vi "tm_trans.vi"(10 "Long":dbl, 11 "Lat":dbl) -> (2 "Numeric":dbl, 3 "out_pt":dbl)   [LabVIEW 2020]
uses:
  <vilib>/imath/engines/lvmath2/RunTimeEngine/Managers/WorkSpace/UID Generator.vi
  <vilib>/imath/engines/lvmath2/RunTimeEngine/RunTimeType/NIMS_RunTimeType_From StrictType (excl LVString).vi
  <instcachedir>/0/NIMS_RunTimeType_From StrictType (excl LVString)_283B1B2000484AAA8744D21CE97EA49F.lvgen/NIMS_RunTimeType_From StrictType (excl LVString)_283B1B2000484AAA8744D21CE97EA49F_000.vi
  <vilib>/imath/engines/lvmath2/RunTimeEngine/LocalVariableDefStatement/MC_LocalVariableDefStatement_Display.vi
  <vilib>/imath/engines/lvmath2/RunTimeEngine/Managers/SymbolTable/Clear UID.vi
  <vilib>/imath/engines/lvmath2/RunTimeEngine/NodeEndStatement/NIMS_NodeEndStatement_Output.vi
  <instcachedir>/0/NIMS_NodeEndStatement_Output_53EC0D466D134D7ABD903AC30B43404B.lvgen/NIMS_NodeEndStatement_Output_53EC0D466D134D7ABD903AC30B43404B_001.vi
  <vilib>/imath/engines/lvmath2/RunTimeEngine/ErrorHandling/NIMS_Finalize Error.vi
  <vilib>/imath/engines/lvmath2/RunTimeEngine/Managers/SymbolTable/NIMS_WorkSpace.lvlib
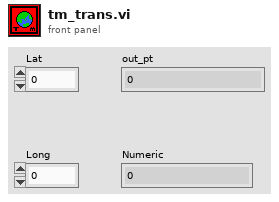
[diagram p1: front panel]
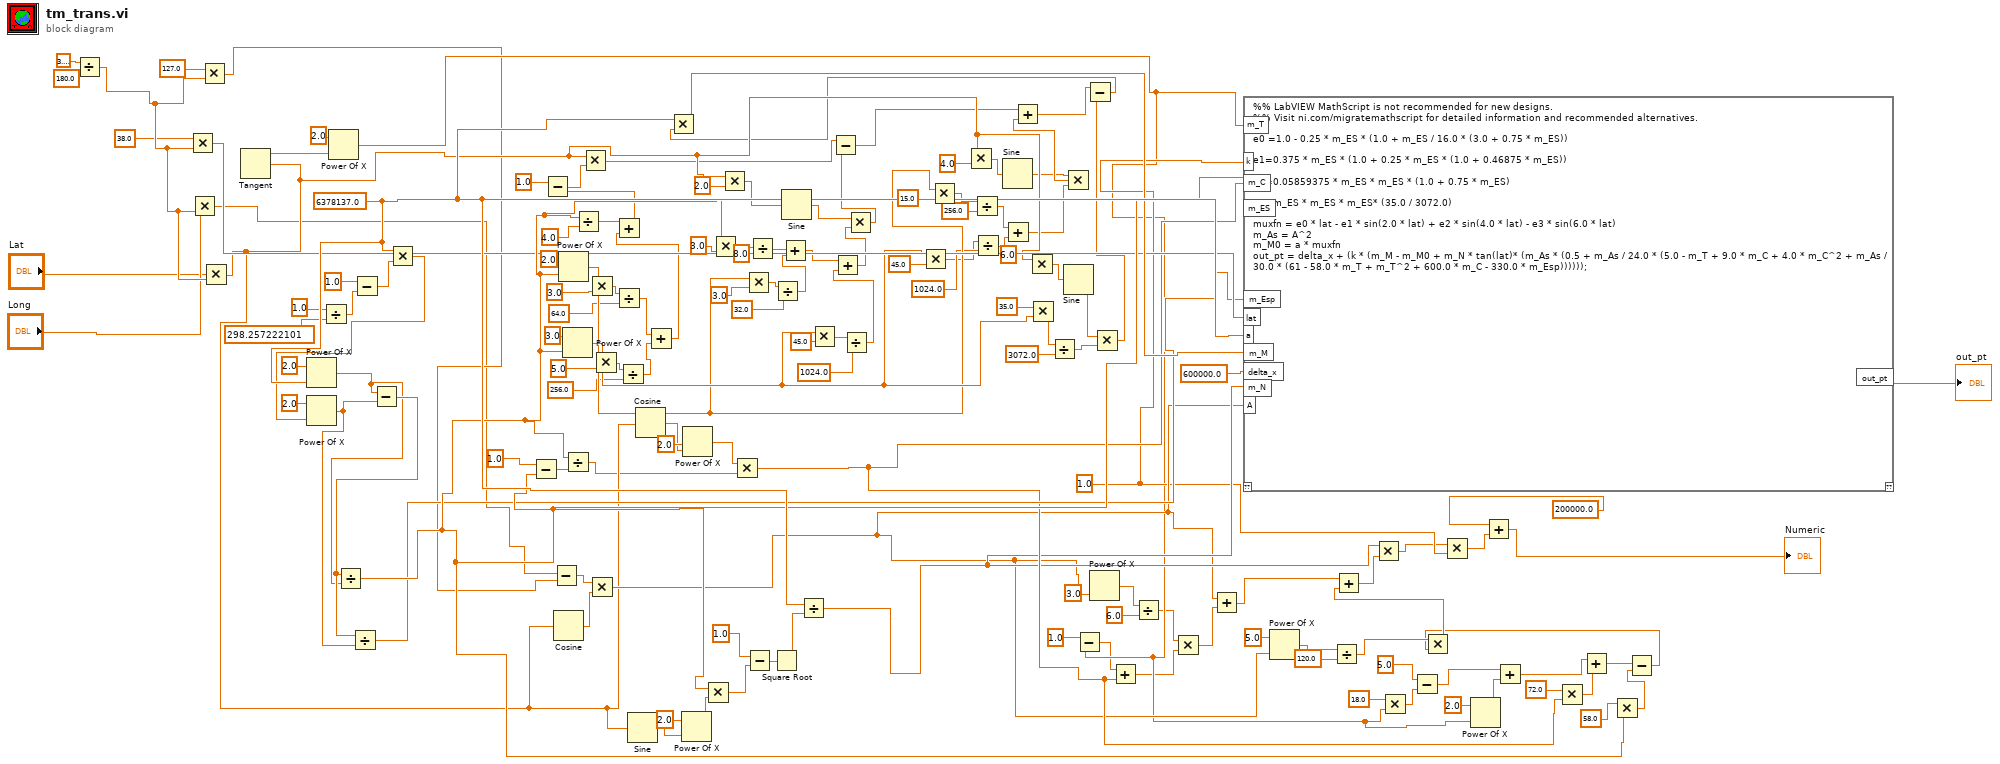
[diagram p0: block diagram]
diagram:
  w133 = 1.0 ("k")
  w143 = 6378137.0
  n1 = Divide(x=3.141592653589793, y=180.0) -> (x/y=w127:dbl)
  n2 = Multiply(x=38.0 ("Latitude0"), y=w127) -> (x*y=w140:dbl)
  n3 = Multiply(x="Long", y=w127) -> (x*y=w129:dbl)
  n4 = Multiply(x=127.0 ("Longtitude0"), y=w127) -> (x*y=w130:dbl)
  n5 = Multiply(x="Lat", y=w127) -> (x*y=w131:dbl)
  n6 = Tangent(1:w131) -> (0:w11:dbl)
  n7 = Power Of X(1:w143, 2:2.0 ("y")) -> (0:w88:dbl)
  n8 = Divide(x=1.0, y=298.257222101) -> (x/y=w6:dbl)
  n9 = Power Of X(1:w11, 2:2.0 ("x")) -> (0:w132:dbl)
  n10 = Subtract(x=1.0, y=w6) -> (x-y=w9:dbl)
  n11 = Multiply(x=w143, y=w9) -> (x*y=w128:dbl)
  n12 = Power Of X(1:w128, 2:2.0 ("y")) -> (0:w90:dbl)
  n13 = Subtract(x=w88, y=w90) -> (x-y=w89:dbl)
  n14 = Divide(x=w89, y=w88) -> (x/y=w141:dbl)
  n15 = Divide(x=w89, y=w90) -> (x/y=w139:dbl)
  n16 = Subtract(x=1.0, y=w141) -> (x-y=w74:dbl)
  n17 = Subtract(x=w129, y=w130) -> (x-y=w80:dbl)
  n18 = Cosine(x=w131) -> (cos(x)=w79:dbl)
  n19 = Power Of X(1:w141, 2:2.0 ("y")) -> (0:w91:dbl)
  n20 = Power Of X(1:w141, 2:3.0 ("y")) -> (0:w92:dbl)
  n21 = Divide(x=w141, y=w74) -> (x/y=w78:dbl)
  n22 = Divide(x=w141, y=4.0) -> (x/y=w26:dbl)
  n23 = Multiply(x=w91, y=3.0) -> (x*y=w17:dbl)
  n24 = Multiply(x=w80, y=w79) -> (x*y=w134:dbl)
  n25 = Multiply(x=w92, y=5.0) -> (x*y=w21:dbl)
  n26 = Divide(x=w17, y=64.0) -> (x/y=w24:dbl)
  n27 = Divide(x=w21, y=256.0) -> (x/y=w23:dbl)
  n28 = Sine(x=w131) -> (sin(x)=w83:dbl)
  n29 = Cosine(x=w131) -> (cos(x)=w75:dbl)
  n30 = Add(x=w24, y=w23) -> (x+y=w25:dbl)
  n31 = Add(x=w26, y=w25) -> (x+y=w27:dbl)
  n32 = Subtract(x=1.0, y=w27) -> (x-y=w29:dbl)
  n33 = Multiply(x=w131, y=w29) -> (x*y=w47:dbl)
  n34 = Power Of X(1:w83, 2:2.0 ("y")) -> (0:w85:dbl)
  n35 = Power Of X(1:w75, 2:2.0 ("y")) -> (0:w77:dbl)
  n36 = Multiply(x=w141, y=w85) -> (x*y=w86:dbl)
  n37 = Multiply(x=w141, y=3.0) -> (x*y=w31:dbl)
  n38 = Multiply(x=w131, y=2.0) -> (x*y=w44:dbl)
  n39 = Multiply(x=w77, y=w78) -> (x*y=w136:dbl)
  n40 = Multiply(x=w91, y=3.0) -> (x*y=w34:dbl)
  n41 = Subtract(x=1.0, y=w86) -> (x-y=w81:dbl)
  n42 = Divide(x=w31, y=8.0) -> (x/y=w37:dbl)
  n43 = Square Root(x=w81) -> (sqrt(x)=w87:dbl)
  n44 = Divide(x=w34, y=32.0) -> (x/y=w36:dbl)
  n45 = Add(x=w37, y=w36) -> (x+y=w42:dbl)
  n46 = Sine(x=w44) -> (sin(x)=w46:dbl)
  n47 = Divide(x=w143, y=w87) -> (x/y=w135:dbl)
  n48 = Multiply(x=w92, y=45.0) -> (x*y=w40:dbl)
  n49 = Divide(x=w40, y=1024.0) -> (x/y=w41:dbl)
  n50 = Add(x=w42, y=w41) -> (x+y=w45:dbl)
  n51 = Multiply(x=w46, y=w45) -> (x*y=w48:dbl)
  n52 = Subtract(x=w47, y=w48) -> (x-y=w61:dbl)
  n53 = Multiply(x=w92, y=45.0) -> (x*y=w53:dbl)
  n54 = Multiply(x=w91, y=15.0) -> (x*y=w50:dbl)
  n55 = Multiply(x=w131, y=4.0) -> (x*y=w58:dbl)
  n56 = Divide(x=w50, y=256.0) -> (x/y=w55:dbl)
  n57 = Divide(x=w53, y=1024.0) -> (x/y=w56:dbl)
  n58 = Sine(x=w58) -> (sin(x)=w59:dbl)
  n59 = Add(x=w55, y=w56) -> (x+y=w60:dbl)
  n60 = Multiply(x=w131, y=6.0) -> (x*y=w67:dbl)
  n61 = Multiply(x=35.0, y=w92) -> (x*y=w64:dbl)
  n62 = Divide(x=w64, y=3072.0) -> (x/y=w66:dbl)
  n63 = Multiply(x=w59, y=w60) -> (x*y=w62:dbl)
  n64 = Add(x=w61, y=w62) -> (x+y=w70:dbl)
  n65 = Sine(x=w67) -> (sin(x)=w68:dbl)
  n66 = Subtract(x=1.0, y=w132) -> (x-y=w96:dbl)
  n67 = Power Of X(1:w134, 2:3.0 ("y")) -> (0:w99:dbl)
  n68 = Multiply(x=w68, y=w66) -> (x*y=w71:dbl)
  n69 = Subtract(x=w70, y=w71) -> (x-y=w72:dbl)
  n70 = Multiply(x=w143, y=w72) -> (x*y=w142:dbl)
  n71 = Add(x=w96, y=w136) -> (x+y=w100:dbl)
  n72 = Divide(x=w99, y=6.0) -> (x/y=w101:dbl)
  n73 = Multiply(x=w101, y=w100) -> (x*y=w102:dbl)
  n74 = Add(x=w134, y=w102) -> (x+y=w121:dbl)
  n75 = mathscript code="%% LabVIEW MathScript is not recommended for new designs.\n%% Visit ni.com/migratemathscript for detailed information and recommended alternatives.\n\ne0 =1.0 - 0.25 * m_ES * (1.0 + m_ES / 16.0 * (3.0 + 0.75 * m_ES))\n\ne1=0.375 * m_ES * (1.0 + 0.25 * m_ES * (1.0 + 0.46875 * m_ES))\n\ne2=0.05859375 * m_ES * m_ES * (1.0 + 0.75 * m_ES)\n\ne3=m_ES * m_ES * m_ES* (35.0 / 3072.0)\n\nmuxfn = e0 * lat - e1 * sin(2.0 * lat) + e2 * sin(4.0 * lat) - e3 * sin(6.0 * lat)\nm_As = A^2\nm_M0 = a * muxfn\nout_pt = delta_x + (k * (m_M - m_M0 + m_N * tan(lat)* (m_As * (0.5 + m_As / 24.0 * (5.0 - m_T + 9.0 * m_C + 4.0 * m_C^2 + m_As / 30.0 * (61 - 58.0 * m_T + m_T^2 + 600.0 * m_C - 330.0 * m_Esp))))));"("k"=w133, "m_ES"=w141, "lat"=w140, "a"=w143, "m_M"=w142, "delta_x"=600000.0 ("delta x"), "m_N"=w135, "A"=w134, "m_T"=w132, "m_C"=w136, "m_Esp"=w139) -> ("out_pt"=→"out_pt":dbl)  [unwired: 1 in, 1 out]
  n76 = Power Of X(1:w134, 2:5.0 ("y")) -> (0:w104:dbl)
  n77 = Divide(x=w104, y=120.0) -> (x/y=w119:dbl)
  n78 = Multiply(x=18.0, y=w132) -> (x*y=w108:dbl)
  n79 = Subtract(x=5.0, y=w108) -> (x-y=w111:dbl)
  n80 = Power Of X(1:w132, 2:2.0 ("y")) -> (0:w110:dbl)
  n81 = Add(x=w111, y=w110) -> (x+y=w114:dbl)
  n82 = Multiply(x=72.0, y=w136) -> (x*y=w115:dbl)
  n83 = Add(x=w114, y=w115) -> (x+y=w117:dbl)
  n84 = Multiply(x=58.0, y=w141) -> (x*y=w116:dbl)
  n85 = Subtract(x=w117, y=w116) -> (x-y=w118:dbl)
  n86 = Multiply(x=w119, y=w118) -> (x*y=w120:dbl)
  n87 = Add(x=w121, y=w120) -> (x+y=w122:dbl)
  n88 = Multiply(x=w135, y=w122) -> (x*y=w123:dbl)
  n89 = Multiply(x=w123, y=w133) -> (x*y=w124:dbl)
  n90 = Add(x=200000.0 ("delta y"), y=w124) -> (x+y=→"Numeric":dbl)
